vi "HEWH Station Timer.vi"(7 "Station ID":T1, 8 "error in (no error)":errorcluster, 10 "Reset Timer (A)":bool, 11 "Reset Timer (Cluster)":bool) -> (0 "error out":errorcluster, 2 "Elapsed Time (sec)- String":string, 3 "Elapsed Time (sec)":dbl)   [LabVIEW 2016]
uses:
  Custom Instrument Control/MW100/Type Definitions/Station ID Selector.ctl
  Utility/Type Definitions/UTILITY Notifier.ctl
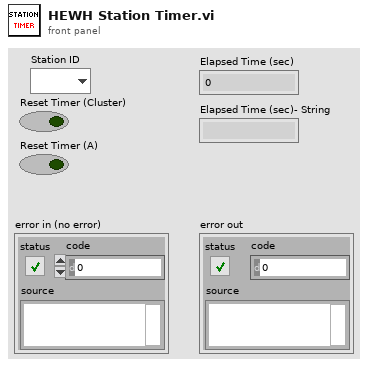
[diagram p1: front panel]
types:
  T1 = typedef "Station ID Selector.ctl" = enum16{"", "A", "B", "C", "D", "Global"}
  T2 = typedef "UTILITY Notifier.ctl" = enum16{"Set", "Read", "Release Ref"}
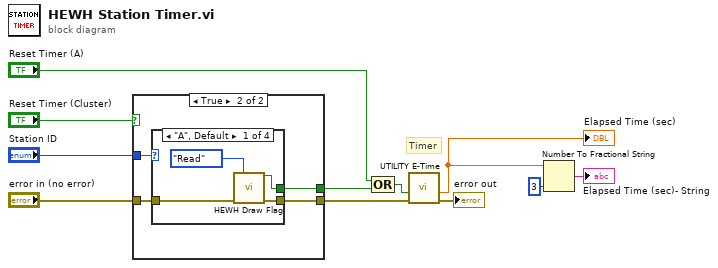
[diagram p0: block diagram]
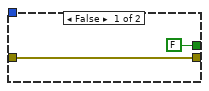
[diagram p2: hidden frame]
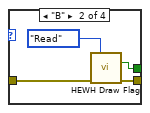
[diagram p3: hidden frame]
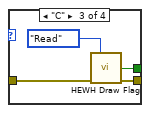
[diagram p4: hidden frame]
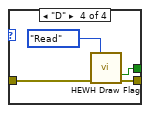
[diagram p5: hidden frame]
diagram:
  # "Timer"
  n1 = case shown="True" "Reset Timer (Cluster)" {
    tunnel: "error in (no error)" -> [w12 w17]
    tunnel: [w12 w16] -> w9
    tunnel: [FALSE ("Station A") w15] -> w10
    tunnel: "Station ID" -> [_ w14]
    frame False {
    }
    frame True {
      n2 = case shown="\"A\", Default" w14 {
        tunnel: w17 -> [w20 w24 w28 w32]
        tunnel: [w19 w23 w27 w31] -> w16
        tunnel: [w18 w22 w26 w30] -> w15
        frame "A", Default {
          n3 = call "HEWH Draw Flag.vi"("Status"=UTILITY_Notifier."Read", "Error In"=w20) -> ("Station A"=w18:bool, "Error Out"=w19:errorcluster)  [unwired: 9 in, 3 out]
        }
        frame "B" {
          n4 = call "HEWH Draw Flag.vi"("Status"=UTILITY_Notifier."Read", "Error In"=w24) -> ("Station B"=w22:bool, "Error Out"=w23:errorcluster)  [unwired: 9 in, 3 out]
        }
        frame "C" {
          n5 = call "HEWH Draw Flag.vi"("Status"=UTILITY_Notifier."Read", "Error In"=w28) -> ("Station C"=w26:bool, "Error Out"=w27:errorcluster)  [unwired: 9 in, 3 out]
        }
        frame "D" {
          n6 = call "HEWH Draw Flag.vi"("Status"=UTILITY_Notifier."Read", "Error In"=w32) -> ("Station D"=w30:bool, "Error Out"=w31:errorcluster)  [unwired: 9 in, 3 out]
        }
      }
    }
  }
  n7 = Compound Arithmetic op=OR("Reset Timer (A)", w10) -> (w7:bool)
  n8 = call "UTILITY E-Time.vi"("error in (no error)"=w9, "Reset"=w7) -> ("error out"=→"error out":errorcluster, "Elapsed Time (sec)"=w2:dbl)  [unwired: 7 in, 1 out]
  "Elapsed Time (sec)" <- w2
  n9 = Number To Fractional String(number=w2, precision (6)=i16 3) -> (F-format string=→"Elapsed Time (sec)- String":string)  [unwired: 2 in]
